vi "HealthCheckHallEffect (1).vi"(1 "Array":dbl[](array[numeric])) -> (0 "Array 2":bool[](array[boolean]))   [LabVIEW 2017]
uses:
  NominalRangeGLOBAL.vi
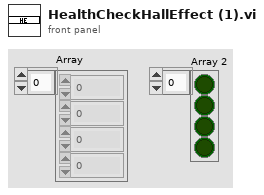
[diagram p1: front panel]
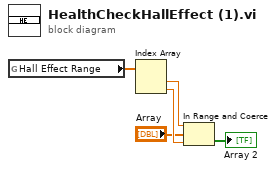
[diagram p0: block diagram]
diagram:
  n1 = global read "NominalRangeGLOBAL.vi" "Hall Effect Range"() -> (w5:dbl[])
  n2 = Index Array(array=w5) -> (element #1=w4:dbl, element #2=w3:dbl)  [unwired: 2 in]
  n3 = In Range and Coerce(upper limit=w4, x="Array", lower limit=w3) -> (In Range?=→"Array 2":bool[])  [unwired: 1 out]
